vi "Testv2.vi"(8 "Cluster In":T2, 9 "Numeric In":i32, 10 "Test In":T1, 11 "LUnit Test Case In":refnum<class "Test Case.lvclass">) -> (0 "Cluster Out":T2, 2 "Test Out":T1, 3 "LUnit Test Case Out":refnum<class "Test Case.lvclass">)   [LabVIEW 2022 SP3]
uses:
  <vilib>/Astemes/LUnit/Test Case.lvclass
  Test.ctl
  Cluster Test.ctl
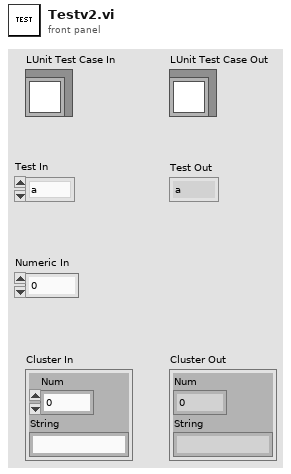
[diagram p1: front panel]
types:
  T1 = typedef "Test.ctl" = enum16{"a", "b"}
  T2 = typedef "Cluster Test.ctl" = cluster{"Num":i32, "String":string}
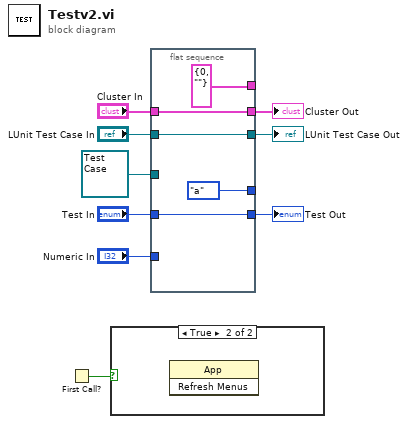
[diagram p0: block diagram]
diagram:
  n1 = First Call?() -> (First Call?: T/F=w7:bool)
  n2 = case shown="True" w7 {
    frame False {
    }
    frame True {
      n3 = invoke class="App" method="Refresh Menus"() -> ()  [unwired: 3 in, 3 out]
    }
  }
  n4 = flat-sequence {
    tunnel: "Cluster In" -> [w14]
    tunnel: [w14] -> w8
    tunnel: "Numeric In" -> [_]
    tunnel: [Test."a"] -> _
    tunnel: [w11] -> w5
    tunnel: [w12] -> w3
    tunnel: "LUnit Test Case In" -> [w12]
    tunnel: refnum<class "Test Case.lvclass"> refnum ("LUnit Test Case In") -> [_]
    tunnel: "Test In" -> [w11]
    tunnel: [T2 {"Num"=0, "String"=""} ("Cluster")] -> _
    frame #0 {
    }
  }
  "Cluster Out" <- w8
  "Test Out" <- w5
  "LUnit Test Case Out" <- w3
